vi "Select First Item.vi"(8 "error in (no error)":errorcluster, 11 "Application Data in":T1) -> (0 "error out":errorcluster, 3 "Application Data out":T1)   [LabVIEW 2017, in "DSF Configuration Utility.lvlib"]
uses:
  DSF Configuration Utility.lvlib
  Main VI/Application Data.ctl
  DSF/Data Sharing Framework Core/DSF Core.lvlibp/DSF Configuration API/Configuration Session.lvclass
  Main VI/View Mode.ctl
panel:
  # "App\nData"
  # "App\nData"
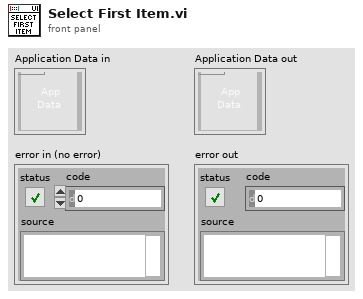
[diagram p1: front panel]
types:
  T1 = typedef "DSF Configuration Utility.lvlib/Application Data.ctl" = cluster{"Item Tree Control":refnum<vi>, "Value Tree Control":refnum<vi>, "DSF Refnum":refnum<class "Configuration Session.lvclass">, "Top-Level VI":refnum<vi>, "View State":T2, "menu reference":refnum<k9>}
  T2 = typedef "DSF Configuration Utility.lvlib/View Mode.ctl" = enum16{"Tree", "List"}
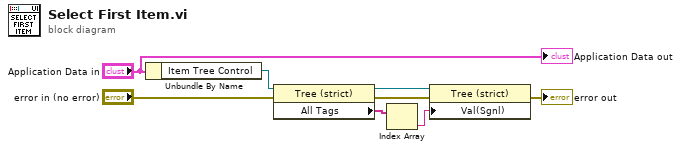
[diagram p0: block diagram]
diagram:
  n1 = Unbundle By Name("Application Data in") -> ("Item Tree Control"=w2:refnum<vi>)
  n2 = property class="Tree (strict)"(reference=w2, error in="error in (no error)") -> (reference out=w4:refnum<vi>, error out=w7:errorcluster, "All Tags"=w3:string[])
  n3 = Index Array(array=w3) -> (element=w5:string)  [unwired: 1 in]
  n4 = property class="Tree (strict)"(reference=w4, error in=w7, "Val(Sgnl)"=w5) -> (error out=→"error out":errorcluster)  [unwired: 1 out]
  "Application Data out" <- "Application Data in"
